vi "Integration Query.vi"(8 "error in (no error)":errorcluster, 9 "Wiring A (0: 1P2W)":u16(ring) items=["1P2W", "1P3W", "3P3W", "3P4W", "3V3A"], 10 "Element":u8=1 min=1 max=6 step=1, 11 "Yokogawa WT1600 in":refnum<class "Yokogawa WT1600.lvclass">) -> (0 "error out":errorcluster, 1 "Integration State":T1, 3 "Yokogawa WT1600 out":refnum<class "Yokogawa WT1600.lvclass">)   [LabVIEW 2014, in "Generic Power Analyzer.lvlib" / "Yokogawa WT1600.lvlib" / "Yokogawa WT1600.lvclass"]
uses:
  Yokogawa WT1600.lvclass
  Universal Power Meter/Universal Power Meter class/Integration State.ctl
panel:
  out "resulting string":string
  out "Integration State 2":string
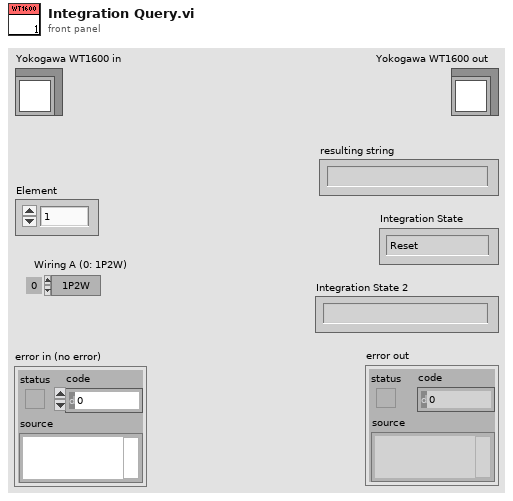
[diagram p1: front panel]
types:
  T1 = typedef "Integration State.ctl" = enum16{"Reset", "Stop", "Start"}
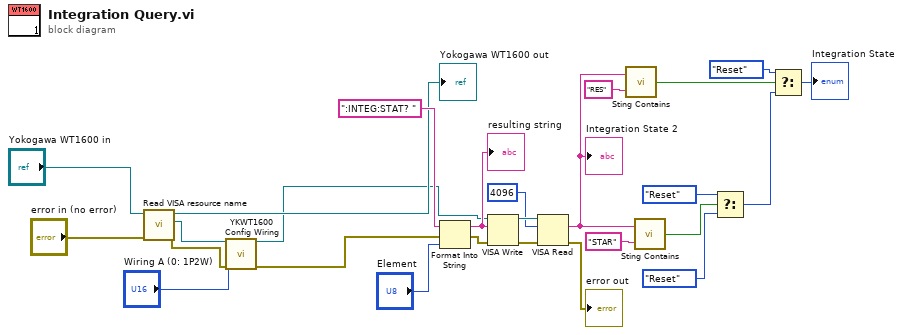
[diagram p0: block diagram]
diagram:
  n1 = call-dynamic "Read VISA resource name.vi"("error in (no error)"="error in (no error)", "Generic Instrument in"="Yokogawa WT1600 in") -> ("error out"=w2:errorcluster, "VISA resource name"=w6:refnum<visa-resource-name>, "Generic Instrument out"=→"Yokogawa WT1600 out":refnum<class "Yokogawa WT1600.lvclass">)  [unwired: 7 in]
  n2 = call <instrlib>:"YKWT1600 Config Wiring.vi"("VISA session"=w6, "Wiring A (0: 1P2W)"="Wiring A (0: 1P2W)", "error in (no error)"=w2) -> ("dup VISA session"=w5:refnum<visa-resource-name>, "error out"=w3:errorcluster)  [unwired: 11 in]
  n3 = Format Into String(initial string=":INTEG:STAT? " ("write buffer"), error in=w3, "Element") -> (resulting string=w21:string, error out=w4:errorcluster)  [unwired: 1 in]
  "resulting string" <- w21
  n4 = VISA Write(VISA resource name=w5, write buffer=w21, error in (no error)=w4) -> (VISA resource name out=w26:refnum<visa-resource-name>, error out=w25:errorcluster)  [unwired: 1 out]
  n5 = VISA Read(VISA resource name=w26, byte count=u32 4096, error in (no error)=w25) -> (read buffer=w12:string, error out=→"error out":errorcluster)  [unwired: 2 out]
  "Integration State 2" <- w12
  n6 = call "Sting Contains.vi"("Expression to evaluate"="RES", "Input String"=w12) -> ("Boolean"=w19:bool)
  n7 = call "Sting Contains.vi"("Expression to evaluate"="STAR", "Input String"=w12) -> ("Boolean"=w17:bool)
  n8 = Select(t=Integration_State."Reset" ("Integration State"), s=w17, f=Integration_State."Reset" ("Integration State")) -> (s? t:f=w16:T1)
  n9 = Select(t=Integration_State."Reset" ("Integration State"), s=w19, f=w16) -> (s? t:f=→"Integration State":T1)
